vi "UpdateDataString.vi"(10 "Display State In":T1, 11 "Data In":T2) -> (1 "Data Changed?":bool, 2 "Display String":string, 3 "lower limit":T2 caption="Data Out")   [LabVIEW 2017, in "Page-XControl.xctl"]
uses:
  Page-XControl.xctl
  Data.ctl
  State.ctl
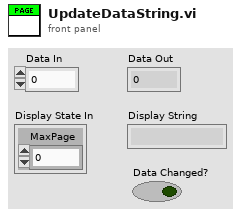
[diagram p1: front panel]
types:
  T1 = typedef "Page-XControl.xctl/State.ctl" = cluster{"MaxPage":u32}
  T2 = typedef "Page-XControl.xctl/Data.ctl" = u32
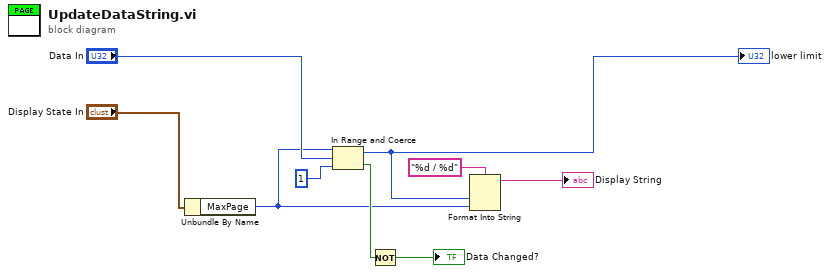
[diagram p0: block diagram]
diagram:
  n1 = Unbundle By Name("Display State In") -> ("MaxPage"=w3:u32)
  n2 = In Range and Coerce(upper limit=w3, x="Data In", lower limit=T2 1) -> (coerced(x)=w6:T2, In Range?=w8:bool)
  "lower limit" <- w6
  n3 = Not(x=w8) -> (.not. x?=→"Data Changed?":bool)
  n4 = Format Into String(format string="%d / %d", w6, w3) -> (resulting string=→"Display String":string)  [unwired: 2 in, 1 out]
